vi "Close Lidar.vi"(8 "error in (no error)":errorcluster, 11 "SerialPortRef":T1) -> (0 "error out":errorcluster)   [LabVIEW 2013]
uses:
  <vilib>/Rock Robotics/WPI/SerialPort/WPI_SerialPortRef.ctl
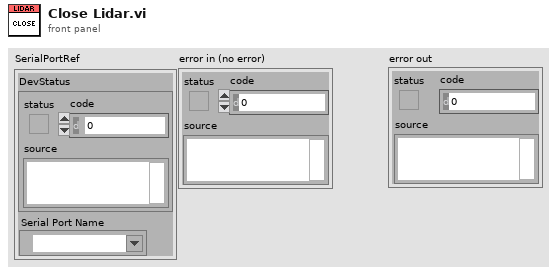
[diagram p1: front panel]
types:
  T1 = typedef "WPI_SerialPortRef.ctl" = cluster{"DevStatus":errorcluster, "Serial Port Name":refnum<visa-resource-name>}
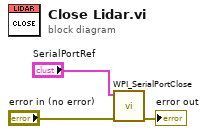
[diagram p0: block diagram]
diagram:
  n1 = call <vilib>:"WPI_SerialPortClose.vi"("error in (no error)"="error in (no error)", "SerialPortRef"="SerialPortRef") -> ("error out"=→"error out":errorcluster)  [unwired: 9 in]
